vi "create data directories.vi"(10 "create directories":path[](array[path]), 11 "root directory":path) -> (2 "directories":path[](array[path]))   [LabVIEW 2013, in "Shared Memory Runtime.lvclass"]
uses:
  Shared Memory Runtime.lvclass
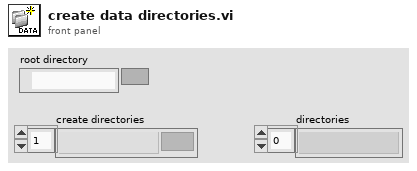
[diagram p1: front panel]
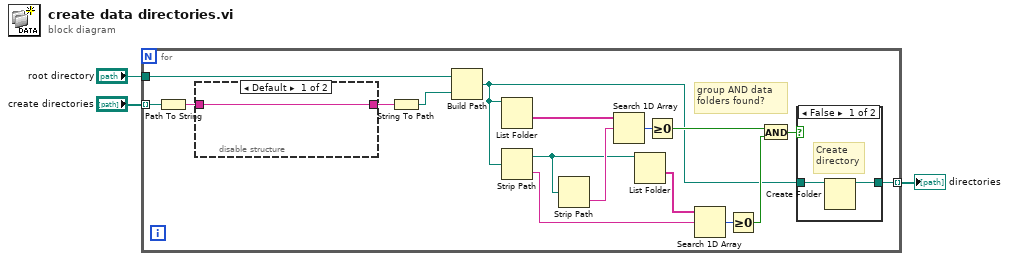
[diagram p0: block diagram]
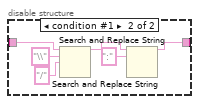
[diagram p2: hidden frame]
diagram:
  n1 = for {
    tunnel: "create directories" -> [w7] mode=indexing
    tunnel: "root directory" -> [w9]
    tunnel: [w8] -> w2 mode=indexing
    # "group AND data \nfolders found?"
    n2 = Path To String(path=w7) -> (string=w6:string)
    n3 = disable-structure shown="Default" {
      disable-tunnel: w6 -> [w21 w25]
      disable-tunnel: [w21 w22] -> w5
      frame condition #0 (active) {
      }
      frame condition #1 {
        n4 = Search and Replace String(input string=w25, search string="\\", replace string="/" ("replace string (\"\")")) -> (result string=w23:string)  [unwired: 5 in, 3 out]
        n5 = Search and Replace String(input string=w23, search string=":") -> (result string=w22:string)  [unwired: 6 in, 3 out]
      }
    }
    n6 = String To Path(string=w5) -> (path=w4:path)
    n7 = Build Path(base path=w9, name or relative path=w4) -> (appended path=w10:path)
    n8 = List Folder(path=w10) -> (folder names=w20:string[])  [unwired: 3 in, 3 out]
    n9 = Strip Path(path=w10) -> (stripped path=w13:path, name=w11:string)
    n10 = Strip Path(path=w13) -> (name=w18:string)  [unwired: 1 out]
    n11 = Search 1D Array(1D array=w20, element=w18) -> (index of element=w19:i32)  [unwired: 1 in]
    n12 = List Folder(path=w13) -> (folder names=w12:string[])  [unwired: 3 in, 3 out]
    n13 = Greater Or Equal To 0?(x=w19) -> (x >= 0?=w16:bool)
    n14 = Search 1D Array(1D array=w12, element=w11) -> (index of element=w17:i32)  [unwired: 1 in]
    n15 = Greater Or Equal To 0?(x=w17) -> (x >= 0?=w15:bool)
    n16 = And(x=w16, y=w15) -> (x .and. y?=w14:bool)
    n17 = case shown="False" w14 {
      tunnel: [w28 w30] -> w8
      tunnel: w10 -> [w29 w30]
      frame False {
        # "Create\ndirectory"
        n18 = Create Folder(path (use dialog)=w29) -> (created path=w28:path)  [unwired: 2 in, 2 out]
      }
      frame True {
      }
    }
  }
  "directories" <- w2
